vi "2022_day12_sub_check_In_Range.vi"(8 "Val Current":i32, 9 "Y":i32, 10 "X":i32, 11 "Playboard":i32[][](array[numeric])) -> (2 "Checkbox":bool)   [LabVIEW 2021]
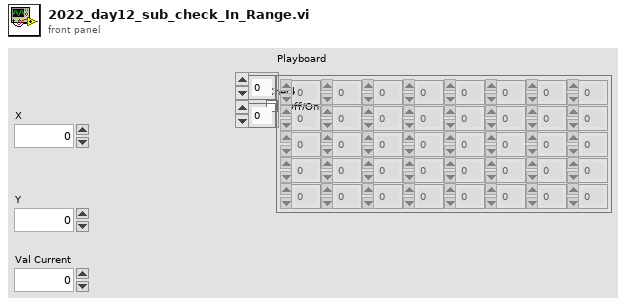
[diagram p1: front panel]
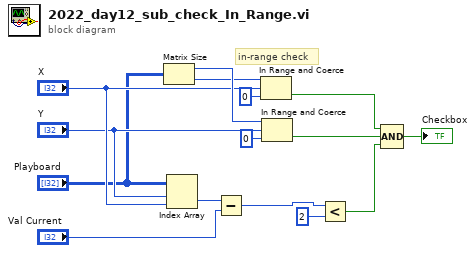
[diagram p0: block diagram]
diagram:
  # "in-range check"
  n1 = Matrix Size(0:"Playboard") -> (1:w10:i32, 2:w9:i32)
  n2 = Index Array(array="Playboard", index (row)="Y", index (col)="X") -> (element=w2:i32)
  n3 = Subtract(x=w2, y="Val Current") -> (x-y=w4:i32)
  n4 = In Range and Coerce(upper limit=w9, x="X", lower limit=0) -> (In Range?=w14:bool)  [unwired: 1 out]
  n5 = In Range and Coerce(upper limit=w10, x="Y", lower limit=0) -> (In Range?=w11:bool)  [unwired: 1 out]
  n6 = Less?(x=w4, y=2) -> (x < y?=w3:bool)
  n7 = Compound Arithmetic op=AND(w14, w11, w3) -> (→"Checkbox":bool)
